vi "Join Five 2 Ten.vi"(0 "OUT 1:0":fxp<+,2,2>, 5 "OUT 1:0 2":fxp<+,2,2>, 7 "OUT 1:0 3":fxp<+,2,2>, 9 "OUT 1:0 4":fxp<+,2,2>, 11 "OUT 1:0 5":fxp<+,2,2>) -> (4 "OUT 9:0":fxp<+,10,10> format="%08b")   [LabVIEW 2019]
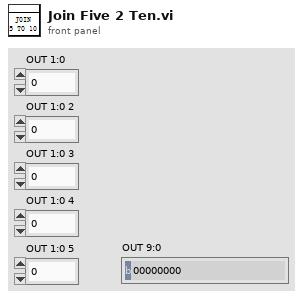
[diagram p1: front panel]
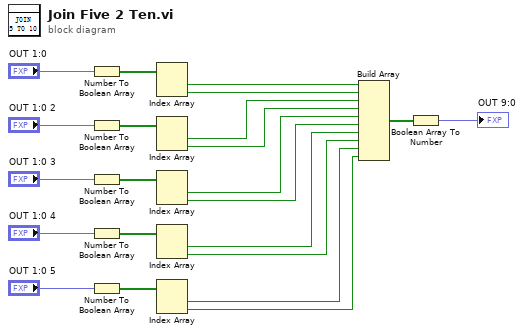
[diagram p0: block diagram]
diagram:
  n1 = Number To Boolean Array(number="OUT 1:0") -> (Boolean array=w17:bool[])
  n2 = Number To Boolean Array(number="OUT 1:0 2") -> (Boolean array=w16:bool[])
  n3 = Number To Boolean Array(number="OUT 1:0 3") -> (Boolean array=w15:bool[])
  n4 = Number To Boolean Array(number="OUT 1:0 4") -> (Boolean array=w14:bool[])
  n5 = Number To Boolean Array(number="OUT 1:0 5") -> (Boolean array=w13:bool[])
  n6 = Index Array(array=w17) -> (element #1=w12:bool, element #2=w11:bool)  [unwired: 2 in]
  n7 = Index Array(array=w16) -> (element #1=w10:bool, element #2=w9:bool)  [unwired: 2 in]
  n8 = Index Array(array=w15) -> (element #1=w8:bool, element #2=w7:bool)  [unwired: 2 in]
  n9 = Index Array(array=w14) -> (element #1=w6:bool, element #2=w5:bool)  [unwired: 2 in]
  n10 = Index Array(array=w13) -> (element #1=w4:bool, element #2=w3:bool)  [unwired: 2 in]
  n11 = Build Array(w12, w11, w10, w9, w8, w7, w6, w5, w4, w3) -> (w2:bool[])
  n12 = Boolean Array To Number(Boolean array=w2) -> (number=→"OUT 9:0":fxp<+,10,10>)
